vi "UpdateDB_PV2.vi"(8 "error in (no error)":errorcluster, 9 "Time Stamp":timestamp, 10 "Double":dbl, 11 "trace ref":refnum<k1>) -> (0 "error out":errorcluster, 3 "trace ref out":refnum<k1>)   [LabVIEW 2013]
uses:
  <vilib>/lvdsc/historical/Write Trace (Numeric).vi
  <vilib>/lvdsc/NI_DSC.lvlib
panel:
  out "x-y":dbl
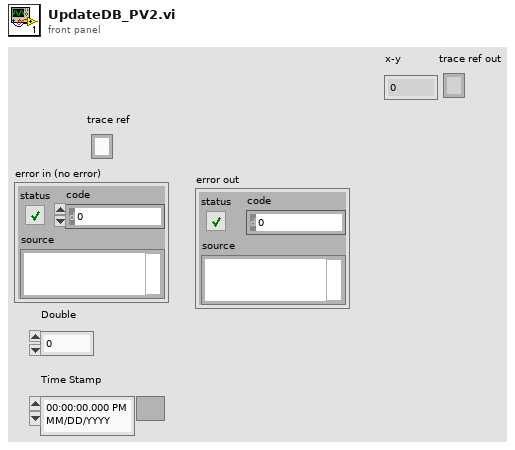
[diagram p1: front panel]
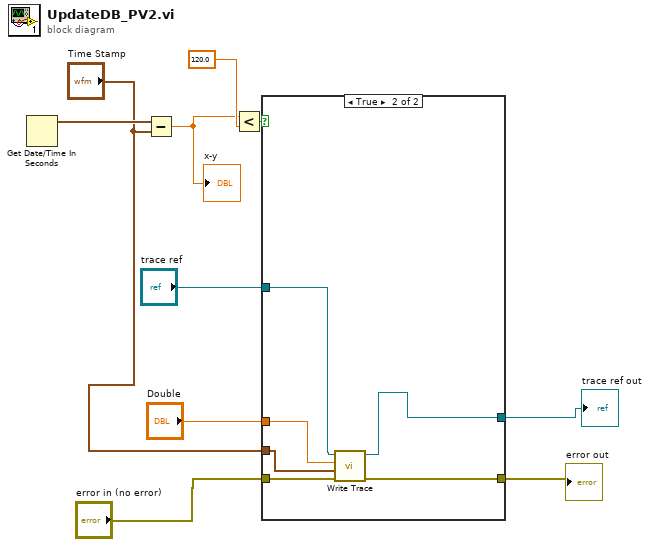
[diagram p0: block diagram]
diagram:
  n1 = Get Date/Time In Seconds() -> (seconds since 1Jan1904=w6:timestamp)
  n2 = Subtract(x=w6, y="Time Stamp") -> (x-y=w7:dbl)
  "x-y" <- w7
  n3 = Less?(x=w7, y=120.0 ("x")) -> (x < y?=w10:bool)
  n4 = case shown="True" w10 {
    tunnel: "error in (no error)" -> [w12 w18]
    tunnel: [w12 w17] -> w1
    tunnel: "Double" -> [_ w16]
    tunnel: "Time Stamp" -> [_ w15]
    tunnel: "trace ref" -> [w11 w14]
    tunnel: [w11 w13] -> w4
    frame False {
    }
    frame True {
      n5 = call-poly <vilib>:"Write Trace.vi"("error in (no error)"=w18, "timestamp (now)"=w15, "value"=w16, "trace ref"=w14) -> ("error out"=w17:errorcluster, "trace ref out"=w13:refnum<k1>)  [unwired: 6 in]
    }
  }
  "error out" <- w1
  "trace ref out" <- w4
